vi "Include Control Ref in Tab.vi"(8 "error in (no error)":errorcluster, 11 "Controls[] in":refnum<vi>[](array[refnum])) -> (0 "error out":errorcluster, 3 "Controls[] out":refnum<vi>[](array[refnum]))   [LabVIEW 2023, in "Label-Driven UI.lvlib"]
uses:
  Label-Driven UI.lvlib
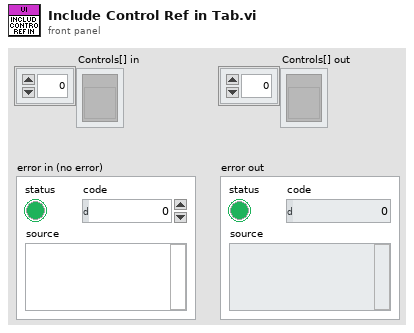
[diagram p1: front panel]
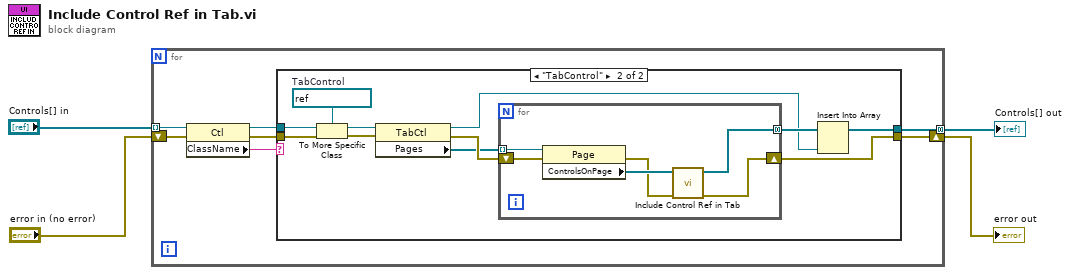
[diagram p0: block diagram]
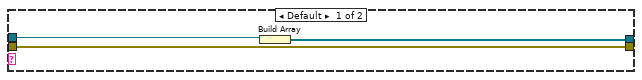
[diagram p2: hidden frame]
diagram:
  n1 = for {
    tunnel: "Controls[] in" -> [w11] mode=indexing
    shift-right: [w6] -> w2
    shift-left: "error in (no error)" -> [w8]
    tunnel: [w5] -> w1 mode=concatenating
    n2 = property class="Ctl"(reference=w11, error in=w8) -> (reference out=w9:refnum<vi>, error out=w7:errorcluster, "ClassName"=w10:string)
    n3 = case shown="\"TabControl\"" w10 {
      tunnel: w9 -> [w14 w25]
      tunnel: w7 -> [w12 w23]
      tunnel: [w13 w16] -> w5
      tunnel: [w12 w18] -> w6
      frame Default {
        n4 = Build Array(w14) -> (w13:refnum<vi>[])
      }
      frame "TabControl" {
        w21 = refnum<vi> refnum  # TabControl
        n5 = To More Specific Class(target class=w21, reference=w25, error in=w23) -> (specific class reference=w24:refnum<vi>, error out=w22:errorcluster)
        n6 = property class="TabCtl"(reference=w24, error in=w22) -> (reference out=w15:refnum<vi>, error out=w20:errorcluster, "Pages"=w19:refnum<vi>[])
        n7 = for {
          shift-right: [w27] -> w18
          shift-left: w20 -> [w30]
          tunnel: w19 -> [w31] mode=indexing
          tunnel: [w26] -> w17 mode=concatenating
          n8 = property class="Page"(reference=w31, error in=w30) -> (error out=w28:errorcluster, "ControlsOnPage"=w29:refnum<vi>[])  [unwired: 1 out]
          n9 = call "Include Control Ref in Tab.vi"("error in (no error)"=w28, "Controls[] in"=w29) -> ("error out"=w27:errorcluster, "Controls[] out"=w26:refnum<vi>[])  [unwired: 8 in]
        }
        n10 = Insert Into Array(array=w17, new element=w15) -> (w16:refnum<vi>[])  [unwired: 1 in]
      }
    }
  }
  "Controls[] out" <- w1
  "error out" <- w2
